vi "Create Observer.vi"(8 "error in (no error)":errorcluster, 11 "Messenger in":refnum<class "Messenger.lvclass">) -> (0 "error out":errorcluster, 2 "Observer":refnum<event-registration>, 3 "Messenger out":refnum<class "Messenger.lvclass">)   [LabVIEW 2015, in "Messenger.lvclass"]
doc: "Creates an observer (User Event) which can be used to receive any messages broadcast by the messenger.\n\nIn practice this VI is used to register a User Event that is used to communicate back to the parent (the process) VI."
uses:
  Messenger.lvclass
  Message/Message.lvclass
  Messenger.lvclass/Messenger.ctl
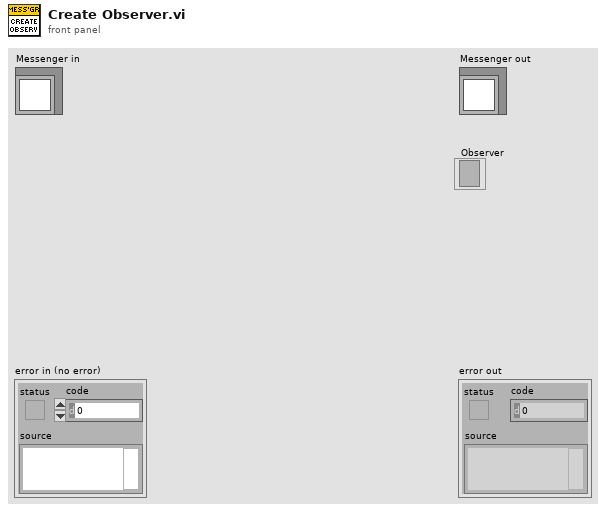
[diagram p1: front panel]
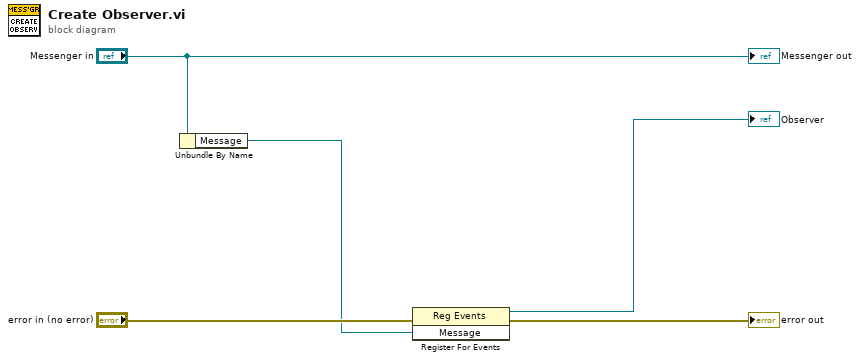
[diagram p0: block diagram]
diagram:
  n1 = Unbundle By Name("Messenger in") -> ("Message"=w1:refnum<user-event>)
  n2 = register-events(error in="error in (no error)", w1) -> (reference out=→"Observer":refnum<event-registration>, error out=→"error out":errorcluster)  [unwired: 1 in]
  "Messenger out" <- "Messenger in"
